vi "initialize_scan.vi"(0 "Scan Directory":string, 5 "Scan Name":string, 9 "Scan Type":string(combo)="New Scan") -> (3 "Path Spec":path, 4 "Path Scan":path, 6 "Number of Spectrometers":i32, 10 "Wrapper Out":u64, 15 "error out":errorcluster)   [LabVIEW 2018]
uses:
  <vilib>/Utility/file.llb/Write Delimited Spreadsheet (string).vi
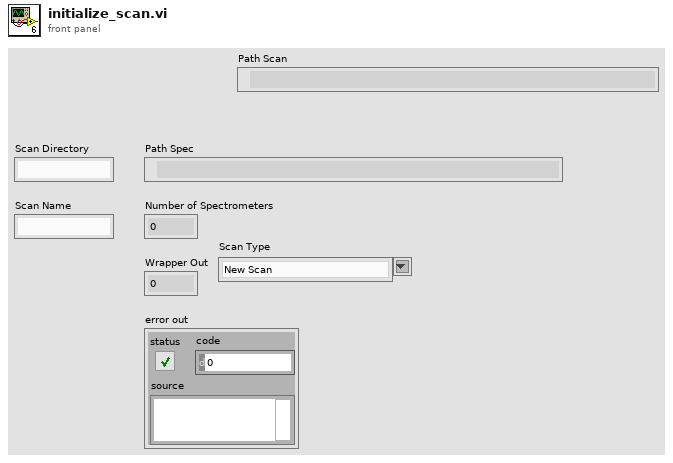
[diagram p1: front panel]
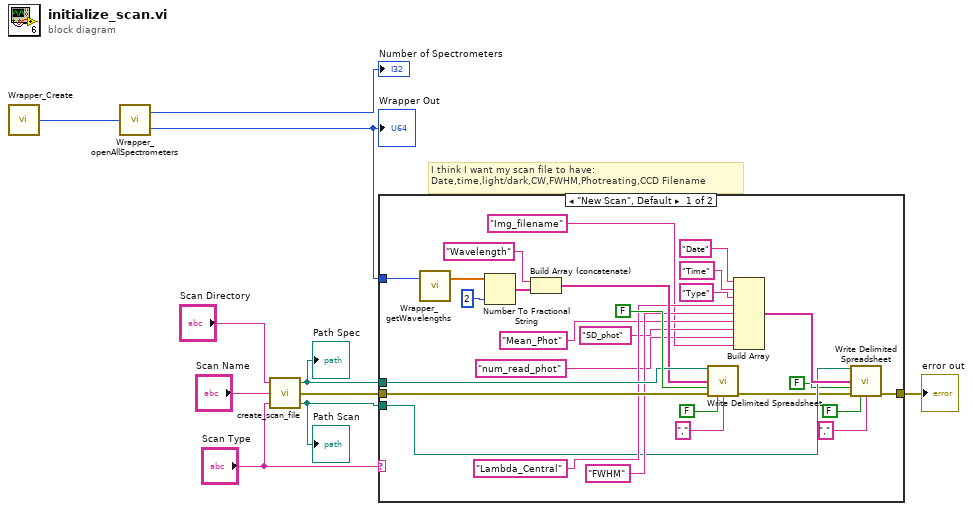
[diagram p0: block diagram]
diagram:
  # "I think I want my scan file to have:\nDate,time,light/dark,CW,FWHM,Photreating,CCD Filename"
  n1 = call "Wrapper_Create.vi"() -> ("Wrapper"=w7:u64)
  n2 = call "Wrapper_openAllSpectrometers.vi"("Wrapper In"=w7) -> ("Number of Spectrometers"=→"Number of Spectrometers":i32, "Wrapper Out"=w5:u64)
  "Wrapper Out" <- w5
  n3 = call "create_scan_file.vi"("Scan Type"="Scan Type", "Scan Name"="Scan Name", "Scan Directory"="Scan Directory") -> ("Path Scan"=w1:path, "Error Out"=w4:errorcluster, "Path Spec"=w6:path)
  "Path Spec" <- w6
  "Path Scan" <- w1
  n4 = case shown="\"New Scan\", Default" "Scan Type" {
    tunnel: w6 -> [w34 _]
    tunnel: w5 -> [w33 _]
    tunnel: w4 -> [w32 w38]
    tunnel: [w14 w38] -> w3
    tunnel: w1 -> [w18 _]
    frame "New Scan", Default {
      n5 = call "Wrapper_getWavelengths.vi"("Wrapper"=w33) -> ("WL Values"=w28:dbl[])  [unwired: 1 in, 1 out]
      n6 = Number To Fractional String(number=w28, precision (6)=i16 2) -> (F-format string=w29:string[])  [unwired: 2 in]
      n7 = Build Array (concatenate)("Wavelength" ("string"), w29) -> (w27:string[])
      n8 = call-poly <vilib>:"Write Delimited Spreadsheet.vi"("file path (dialog if empty)"=w34, "1D data"=w27, "append to file? (new file:F)"=FALSE, "error in (no error)"=w32, "transpose? (no:F)"=FALSE, "delimiter (\\t)"="," ("delimiter (\\t)")) -> ("error out"=w15:errorcluster)  [unwired: 8 in, 1 out]
      n9 = Build Array("Date", "Time" ("element"), "Type" ("element"), "Lambda_Central" ("element"), "FWHM" ("element"), "Mean_Phot" ("element"), "SD_phot" ("element"), "num_read_phot" ("element"), "Img_filename" ("element")) -> (w19:string[])
      n10 = call-poly <vilib>:"Write Delimited Spreadsheet.vi"("file path (dialog if empty)"=w18, "1D data"=w19, "append to file? (new file:F)"=FALSE, "error in (no error)"=w15, "transpose? (no:F)"=FALSE, "delimiter (\\t)"="," ("delimiter (\\t)")) -> ("error out"=w14:errorcluster)  [unwired: 8 in, 1 out]
    }
    frame "Resume Scan" {
    }
  }
  "error out" <- w3
